vi "add line to table.vi"(8 "error in":errorcluster, 10 "line":T1, 11 "operations table":T2) -> (0 "error out":errorcluster)   [LabVIEW 2013, in "alarms module editor node.lvclass"]
uses:
  alarms module editor node.lvclass
  table reference.ctl
  table line.ctl
  <vilib>/NI/Tag Bus Module Framework/channel/TBM channel.lvclass
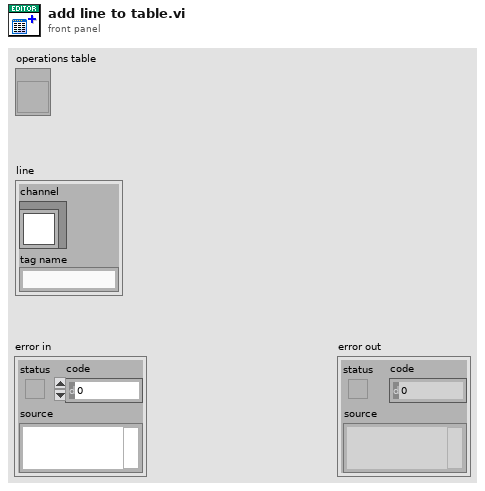
[diagram p1: front panel]
types:
  T1 = typedef "alarms module editor node.lvclass/table line.ctl" = cluster{"channel":refnum<class "TBM channel.lvclass">, "tag name":string}
  T2 = typedef "alarms module editor node.lvclass/table reference.ctl" = refnum<vi>
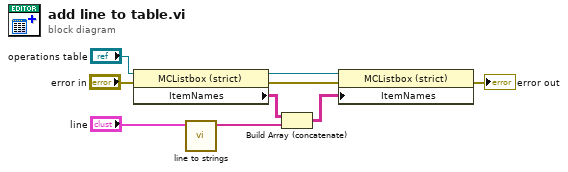
[diagram p0: block diagram]
diagram:
  n1 = property class="MCListbox (strict)"(reference="operations table", error in="error in") -> (reference out=w3:T2, error out=w4:errorcluster, "ItemNames"=w5:string[][])
  n2 = call "line to strings.vi"("line"="line") -> ("strings"=w6:string[])  [unwired: 10 in]
  n3 = Build Array (concatenate)(w5, w6) -> (w2:string[][])
  n4 = property class="MCListbox (strict)"(reference=w3, error in=w4, "ItemNames"=w2) -> (error out=→"error out":errorcluster)  [unwired: 1 out]
